vi "FindPropertyValue.vi"(10 "property":string, 11 "rows":string) -> (3 "value":string)   [LabVIEW 2019]
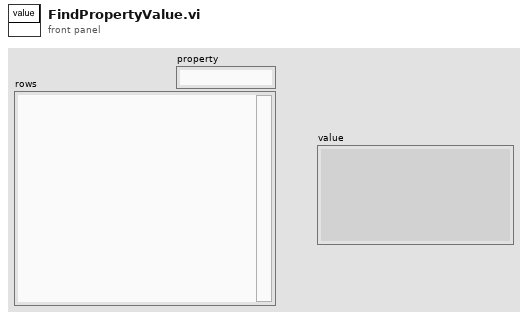
[diagram p1: front panel]
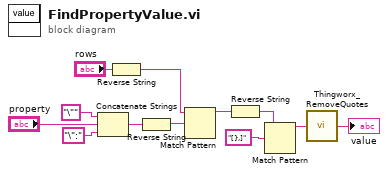
[diagram p0: block diagram]
diagram:
  n1 = Concatenate Strings("\"" ("string"), "property", "\":" ("string")) -> (w8:string)
  n2 = Reverse String(1:"rows") -> (0:w4:string)
  n3 = Reverse String(1:w8) -> (0:w3:string)
  n4 = Match Pattern(string=w4, regular expression=w3) -> (before substring=w2:string)  [unwired: 1 in, 3 out]
  n5 = Reverse String(1:w2) -> (0:w1:string)
  n6 = Match Pattern(string=w1, regular expression="[},]") -> (before substring=w10:string)  [unwired: 1 in, 3 out]
  n7 = call "Thingworx_RemoveQuotes.vi"("Incoming string in"=w10) -> ("Incoming string out"=→"value":string)
